vi "FTW-Logger-Construct.vi"(0 "Initialization Sequence":string, 5 "Logger Configuration":string, 11 "error in":errorcluster) -> (4 "FTW Logger":refnum<class "FTW-Logger-Core.lvclass">, 6 "Incoming Requests":refnum<event-registration>, 15 "error out":errorcluster)   [LabVIEW 2013, in "FTW-Actor.lvlib" / "FTW-Logger-Core.lvclass"]
uses:
  FTW-Logger-Core.lvclass
  Message/Request/FTW-Message-IncomingRequest.lvclass
  Core/src/Time/FTW-Time-DisplayFormat-Timestamp.ctl
  FTW-Logger-Core.lvclass/FTW-Logger-Core.ctl
  Core/utils/CodeGen/JSON Deserialize/FTW-JSON-Deserialize.xnode
  Core/src/Reflection/FTW-Reflection-Type.vi
  Core/src/JSON/FTW-JSON-Core-GetFlattenedValue.vi
  Core/src/JSON/FTW-JSON-Core-LibraryFilepath.vi
  Core/src/JSON/FTW-JSON-Core-LibraryError.vi
panel:
  # "Inputs"
  # "Outputs"
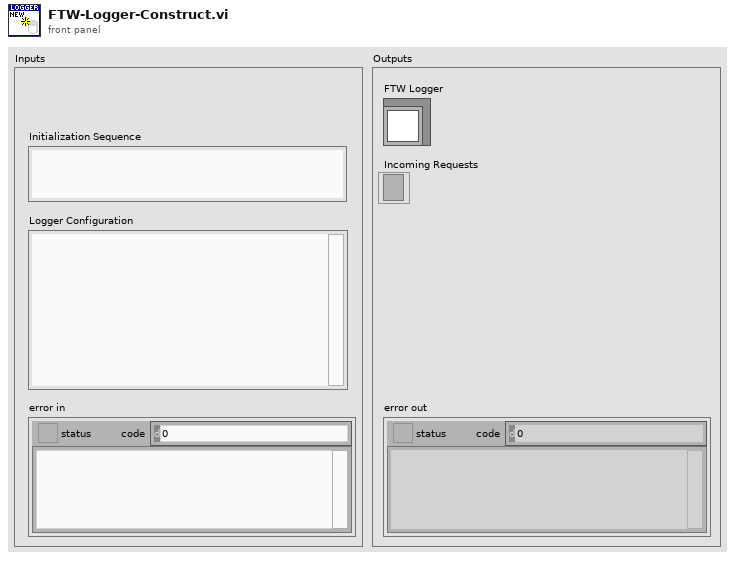
[diagram p1: front panel]
types:
  T1 = typedef "FTW-Time-DisplayFormat-Timestamp.ctl" = enum16{"YYYY-MM-DDT00:00:00.000Z (ISO-8601)", "YYYY-MM-DDT00-00-00Z (Simple ISO-8601)", "YYYY-MM-DD"}
  T2 = cluster{"ApplicationName":string, "LoggerName":string, "LoggerDirectory":path, "LoggerDiskThrashDelay":u32}
  T3 = cluster{"LoggerDirectory":string, "LoggerDiskThrashDelay":u32, "LoggerName":string, "ApplicationName":string}
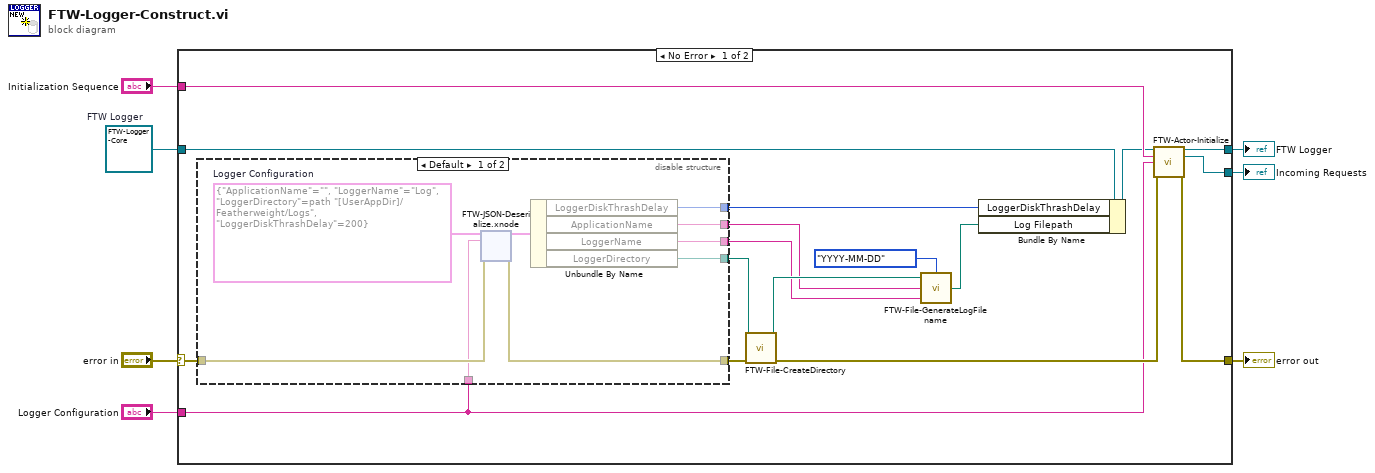
[diagram p0: block diagram]
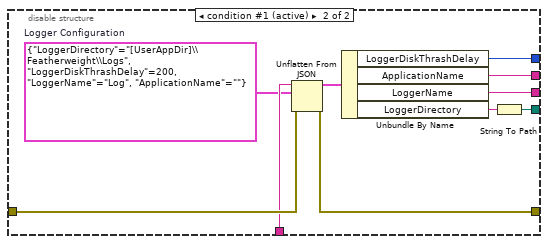
[diagram p2: hidden frame]
diagram:
  w7 = refnum<class "FTW-Logger-Core.lvclass"> refnum  # FTW Logger
  n1 = case shown="No Error" "error in" {
    selector: "error in" -> [w10 w79]
    tunnel: [w22 w79] -> w5
    tunnel: [w24 w78] -> w1
    tunnel: w7 -> [w20 w78]
    tunnel: "Logger Configuration" -> [w8 _]
    tunnel: [w23 _] -> w3
    tunnel: "Initialization Sequence" -> [w21 _]
    frame No Error {
      n2 = disable-structure shown="Default" {
        disable-tunnel: [w33 w77] -> w18
        disable-tunnel: [w32 w76] -> w15
        disable-tunnel: [w31 w75] -> w14
        disable-tunnel: [w30 w71] -> w13
        disable-tunnel: w10 -> [w29 w73]
        disable-tunnel: [w28 w72] -> w9
        disable-tunnel: w8 -> [w27 w70]
        frame condition #0 {
          w26 = T2 {"ApplicationName"="", "LoggerName"="Log", "LoggerDirectory"=path "[UserAppDir]/Featherweight/Logs", "LoggerDiskThrashDelay"=200}  # Logger Configuration
          n3 = xnode "FTW-JSON-Deserialize.xnode"("Type and Defaults"=w26, "JSON String"=w27, "error in"=w29) -> ("Values"=w25:T2, "error out"=w28:errorcluster)
          n4 = Unbundle By Name(w25) -> ("LoggerDiskThrashDelay"=w33:u32, "ApplicationName"=w32:string, "LoggerName"=w31:string, "LoggerDirectory"=w30:path)
        }
        frame condition #1 (active) {
          w69 = T3 {"LoggerDirectory"="[UserAppDir]\\Featherweight\\Logs", "LoggerDiskThrashDelay"=200, "LoggerName"="Log", "ApplicationName"=""}  # Logger Configuration
          n5 = Unflatten From JSON(JSON string=w70, type and defaults=w69, error in (no error)=w73) -> (value=w68:T3, error out=w72:errorcluster)  [unwired: 4 in]
          n6 = Unbundle By Name(w68) -> ("LoggerDiskThrashDelay"=w77:u32, "ApplicationName"=w76:string, "LoggerName"=w75:string, "LoggerDirectory"=w74:string)
          n7 = String To Path(string=w74) -> (path=w71:path)
        }
      }
      n8 = call "FTW-File-CreateDirectory.vi"("Directory to Create"=w13, "error in"=w9) -> ("Created Directory"=w16:path, "error out"=w11:errorcluster)  [unwired: 12 in]
      n9 = call "FTW-File-GenerateLogFilename.vi"("Date Format"=FTW-Time-DisplayFormat-Timestamp."YYYY-MM-DD", "Type"=w14, "Application"=w15, "Directory"=w16) -> ("Filepath"=w12:path)
      n10 = Bundle By Name(cluster=w20, "LoggerDiskThrashDelay"=w18, "Log Filepath"=w12) -> (w19:refnum<class "FTW-Logger-Core.lvclass">)
      n11 = call-dynamic "FTW-Actor-Initialize.vi"("FTW Actor Instance Type"=w19, "Initialization Job Sequence"=w21, "Actor Instance Configuration"=w8, "error in"=w11) -> ("FTW Actor Instance"=w24:refnum<class "FTW-Logger-Core.lvclass">, "Incoming Requests"=w23:refnum<event-registration>, "error out"=w22:errorcluster)  [unwired: 9 in]
    }
    frame Error {
    }
  }
  "error out" <- w5
  "FTW Logger" <- w1
  "Incoming Requests" <- w3
